vi "Write.vi"(0 "System Interface":refnum<class "System Interface.lvclass">, 1 "Terminal":string="Output", 5 "Process Data":T1, 11 "Error In":errorcluster) -> (4 "System Interface out":refnum<class "System Interface.lvclass">, 15 "Error Out":errorcluster)   [LabVIEW 2020, in "ADAS_Data_Type_Template.lvlib"]
uses:
  ADAS_Data_Type_Template.lvlib
  <vilib>/FlexLogger/SDK/PluginSDK.lvlibp/PEFClasses/SDK/System Interface/System Interface.lvclass
  Process Data.ctl
  414300ae-2f3d-445e-aeca-488e23f625b8.vi
  414300ae-2f3d-445e-aeca-488e23f625b8.vi/409c1e6a-7c9d-40e3-aeb2-a56b28beb7cd.vi
  414300ae-2f3d-445e-aeca-488e23f625b8.vi/c12f0ec1-a61b-4634-8df9-4ec1f5a6330b.vi
  414300ae-2f3d-445e-aeca-488e23f625b8.vi/409c1e6a-7c9d-40e3-aeb2-a56b28beb7cd.vi/55125485-cdad-4f1d-89b9-9bdf3801ca7d.vi
  414300ae-2f3d-445e-aeca-488e23f625b8.vi/409c1e6a-7c9d-40e3-aeb2-a56b28beb7cd.vi/c67d7082-f268-4082-9be0-83b0132da06c.vi
  414300ae-2f3d-445e-aeca-488e23f625b8.vi/409c1e6a-7c9d-40e3-aeb2-a56b28beb7cd.vi/1adf875c-fde0-460e-a784-90d221d44610.vi
  414300ae-2f3d-445e-aeca-488e23f625b8.vi/409c1e6a-7c9d-40e3-aeb2-a56b28beb7cd.vi/ef5cfb74-7e3c-4ca5-99ab-4d3670a506f3.vi
  <vilib>/ADAS Record/IODataPEF/Error/Error_CheckAndSetDllError.vi
  <vilib>/ADAS Record/IODataPEF/Error/Error_SetError.vi
  <vilib>/ADAS Record/IODataPEF/CfgMgr/GetPEFConfiguration_DefaultFlatFormat.vi
  <vilib>/ADAS Record/pefCommon/Tracing/SendGenericEvent.vi
  <vilib>/ADAS Record/CustomData/_Custom_RegisterType.vi
  <vilib>/ADAS Record/IODataPEF/Error/ErrorMgr.vi
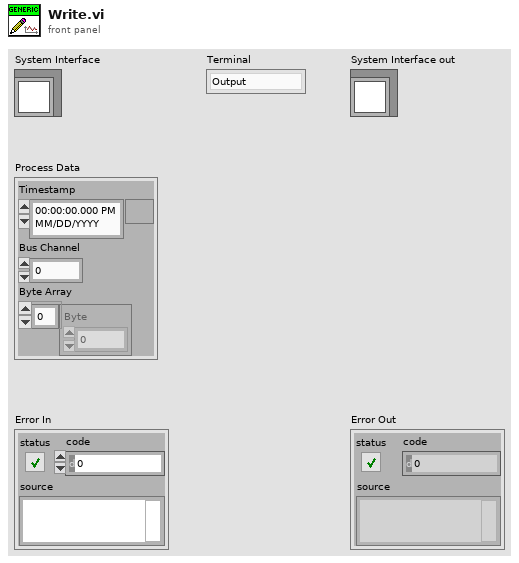
[diagram p1: front panel]
types:
  T1 = typedef "ADAS_Data_Type_Template.lvlib/Process Data.ctl" = cluster{"Timestamp":timestamp, "Bus Channel":u16, "Byte Array":u8[]}
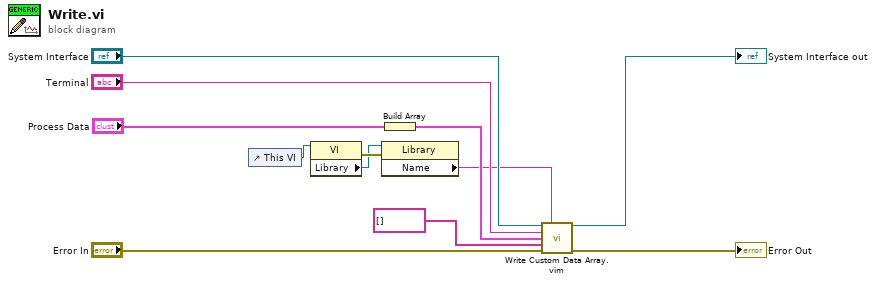
[diagram p0: block diagram]
diagram:
  n1 = control-ref of="This VI"() -> (w5:refnum<vi>)
  n2 = property class="VI"(reference=w5) -> (error out=w4:errorcluster, "Library"=w3:refnum<vi>)  [unwired: 1 in, 1 out]
  n3 = property class="Library"(reference=w3, error in=w4) -> ("Name"=w2:string)  [unwired: 2 out]
  n4 = Build Array("Process Data") -> (w7:T1[])
  n5 = call "Write Custom Data Array.vim"("System Interface"="System Interface", "Type"=w2, "Terminal"="Terminal", "Data"=w7, "Metadata"=string[] [], "error in (no error)"="Error In") -> ("System Interface out"=→"System Interface out":refnum<class "System Interface.lvclass">, "error out"=→"Error Out":errorcluster)  [unwired: 8 in]
